vi "1-2_UnifiedCameraCalibration.vi"() -> ()   [LabVIEW 2016]
uses:
  <vilib>/vision/NI_Vision_Development_Module.lvlib
  <vilib>/vision/Image Controls.llb/IMAQ Image.ctl
panel:
  in  "Boolean":bool
  in  "Path":path
  out "histogram":u32[](array[numeric])
  out "Result Uncertainty":dbl
  out "Result":dbl
  in  "Method":T1(ring)
  out "error out":errorcluster
  in  "error in (no error)":errorcluster
  out "Image Out":T2
  in  "Image In":T2
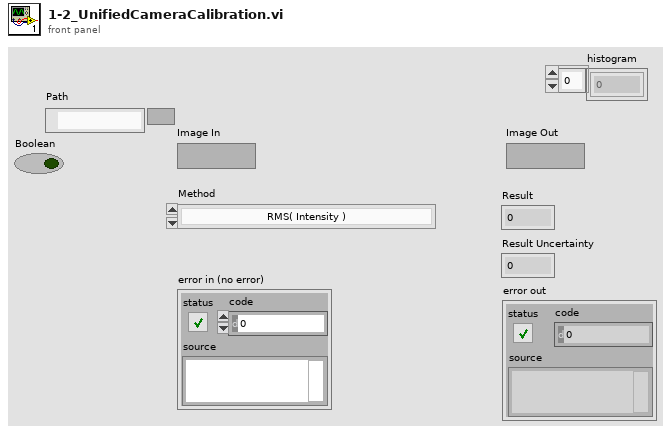
[diagram p1: front panel]
types:
  T1 = enum16{"RMS( Intensity )", "Mean( Laplacian Convolution )"}
  T2 = typedef "IMAQ Image.ctl" = refnum<image>
  T3 = cluster{"histogram":u32[], "Minimal Value":sgl, "Maximal Value":sgl, "Starting Value":sgl, "Interval Width":sgl, "Mean Value":sgl, "Standard  Variation":sgl, "Area (pixels)":i32}
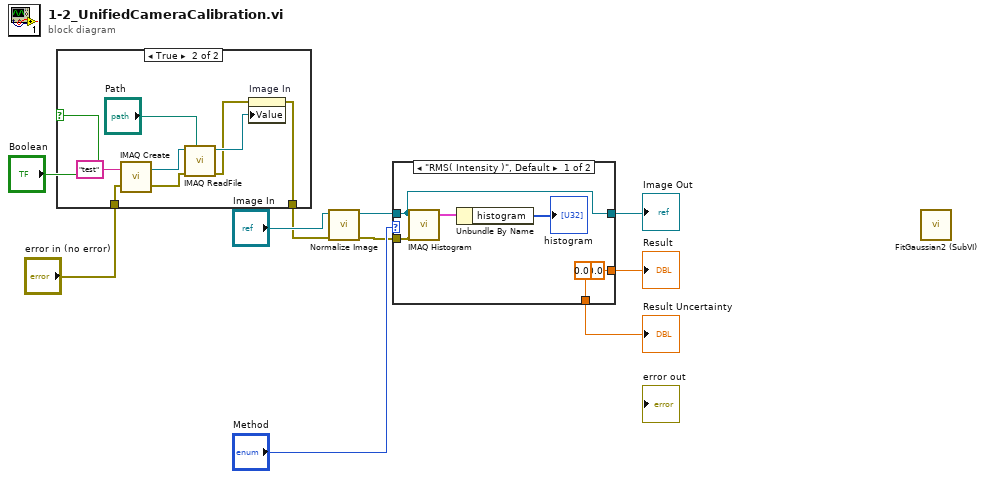
[diagram p0: block diagram]
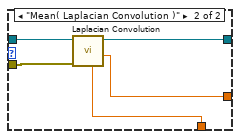
[diagram p3: hidden frame]
diagram:
  n1 = case shown="True" "Boolean" {
    tunnel: [_ w14] -> w3
    tunnel: "error in (no error)" -> [_ w11]
    frame False {
    }
    frame True {
      n2 = call "IMAQ Create"("Image Name"="test", "error in (no error)"=w11) -> ("New Image"=w18:T2, "error out"=w12:errorcluster)  [unwired: 3 in]
      n3 = call "IMAQ ReadFile"("File Path"="Path", "error in (no error)"=w12, "Image"=w18) -> ("error out"=w13:errorcluster, "Image Out"=w16:T2)  [unwired: 4 in, 3 out]
      n4 = property on="Image In" class="IMAQImage (strict)"(error in=w13, "Value"=w16) -> (error out=w14:errorcluster)  [unwired: 1 in, 1 out]
    }
  }
  n5 = call "Normalize Image.vi"("error in (no error)"=w3, "Image In"="Image In") -> ("error out"=w7:errorcluster, "Image Out"=w8:T2)  [unwired: 8 in]
  n6 = case shown="\"RMS( Intensity )\", Default" "Method" {
    tunnel: w8 -> [w19 w29]
    tunnel: w7 -> [w24 w28]
    tunnel: [w19 w27] -> w6
    tunnel: [sgl 0.0 ("Standard  Variation") w26] -> w5
    tunnel: [sgl 0.0 ("Mean Value") w25] -> w4
    frame "RMS( Intensity )", Default {
      n7 = call "IMAQ Histogram"("error in (no error)"=w24, "Image"=w19) -> ("Histogram Report"=w23:T3)  [unwired: 8 in, 1 out]
      n8 = Unbundle By Name(w23) -> ("histogram"=→"histogram":u32[])
    }
    frame "Mean( Laplacian Convolution )" {
      n9 = call "Laplacian Convolution.vi"("error in (no error)"=w28, "Refnum in"=w29) -> ("Mean Value"=w25:sgl, "Refnum out"=w27:T2, "Standard  Variation"=w26:sgl)  [unwired: 4 in, 3 out]
    }
  }
  "Image Out" <- w6
  "Result" <- w4
  "Result Uncertainty" <- w5
  n10 = call "FitGaussian2 (SubVI).vi"() -> ()  [unwired: 14 in, 6 out]
